vi "MoveAwayFromBallSkill.vi"(8 "error in (no error)":errorcluster, 9 "Game in":refnum<class "Game.lvclass">, 10 "Robot":refnum<class "Robot.lvclass">, 11 "MoveAwayFromBallSkill in":refnum<class "MoveAwayFromBallSkill.lvclass">) -> (0 "error out":errorcluster, 2 "Robot out":refnum<class "Robot.lvclass">, 3 "MoveAwayFromBallSkill out":refnum<class "MoveAwayFromBallSkill.lvclass">)   [LabVIEW 2023, in "MoveAwayFromBallSkill.lvclass"]
uses:
  MoveAwayFromBallSkill.lvclass
  Robot_class/Robot.lvclass
  C:/Users/lucio/Desktop/roboime/SSL_AI/Object_class/Object.lvclass
  Game_class/Game.lvclass
  Game_class/Game.lvclass/Game.ctl
  Parameters_class/Parameters.lvclass/Parameters.ctl
  Object_class/Object.lvclass/Object.ctl
  Robot_class/Robot.lvclass/Robot.ctl
  <vilib>/Analysis/baseanly.llb/Unit Vector (DBL).vi
  Object_class/Read position(x,y).vi
  Game_class/Read Parameters.lvclass.vi
  Game_class/Read BallRef.vi
  Parameters_class/Read DistanceStop.vi
  Robot_class/Write dest_x.vi
  Robot_class/Write dest_y.vi
  Robot_class/Write dest_orientation.vi
  Ball_class/Ball.lvclass
  Parameters_class/Parameters.lvclass
  <vilib>/Analysis/NI_AALBase.lvlib
  Utilities_class/Utilities.lvclass
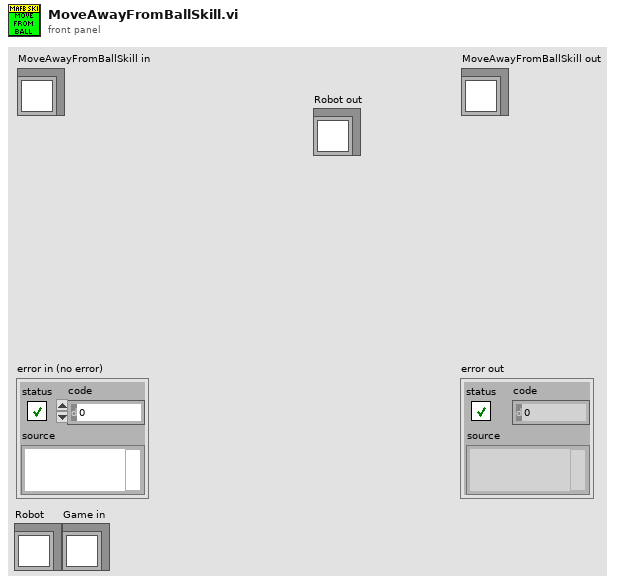
[diagram p1: front panel]
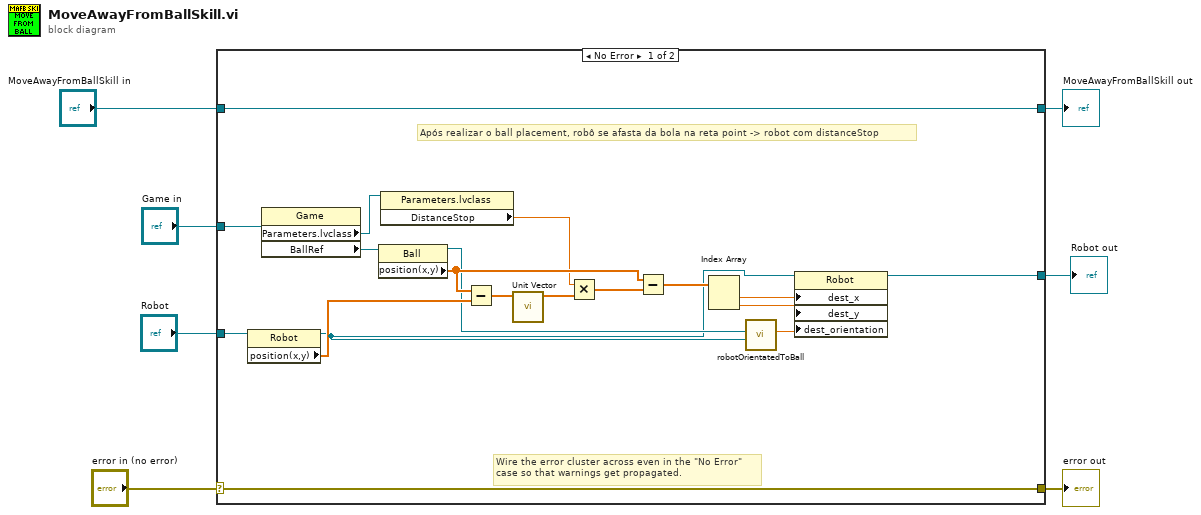
[diagram p0: block diagram]
diagram:
  n1 = case shown="No Error" "error in (no error)" {
    selector: "error in (no error)" -> [w25 w28]
    tunnel: [w25 w28] -> w6
    tunnel: [w26 w27] -> w4
    tunnel: "MoveAwayFromBallSkill in" -> [w26 w27]
    tunnel: "Game in" -> [w24 _]
    tunnel: "Robot" -> [w15 _]
    tunnel: [w11 _] -> w1
    frame No Error {
      # "Após realizar o ball placement, robô se afasta da bola na reta point -> robot com distanceStop"
      # "Wire the error cluster across even in the \"No Error\"\ncase so that warnings get propagated."
      n2 = property class="Robot"(reference=w15) -> (reference out=w8:refnum<class "Robot.lvclass">, "position(x,y)"=w22:dbl[])  [unwired: 1 in, 1 out]
      n3 = property class="Game"(reference=w24) -> ("Parameters.lvclass"=w18:refnum<class "Parameters.lvclass">, "BallRef"=w23:refnum<class "Ball.lvclass">)  [unwired: 1 in, 2 out]
      n4 = property class="Ball"(reference=w23) -> (reference out=w9:refnum<class "Ball.lvclass">, "position(x,y)"=w21:dbl[])  [unwired: 1 in, 1 out]
      n5 = property class="Parameters.lvclass"(reference=w18) -> ("DistanceStop"=w17:dbl)  [unwired: 1 in, 2 out]
      n6 = Subtract(x=w21, y=w22) -> (x-y=w20:dbl[])
      n7 = call-poly <vilib>:"Unit Vector.vi"("Input Vector"=w20) -> ("Unit Vector"=w19:dbl[])  [unwired: 8 in, 2 out]
      n8 = Multiply(x=w17, y=w19) -> (x*y=w16:dbl[])
      n9 = Subtract(x=w21, y=w16) -> (x-y=w14:dbl[])
      n10 = Index Array(array=w14) -> (element #1=w13:dbl, element #2=w12:dbl)  [unwired: 2 in]
      n11 = call "robotOrientatedToBall.vi"("Robot"=w8, "BallRef"=w9) -> ("Orientation"=w10:dbl)  [unwired: 7 in, 2 out]
      n12 = property class="Robot"(reference=w8, "dest_x"=w13, "dest_y"=w12, "dest_orientation"=w10) -> (reference out=w11:refnum<class "Robot.lvclass">)  [unwired: 1 in, 1 out]
    }
    frame Error {
    }
  }
  "error out" <- w6
  "MoveAwayFromBallSkill out" <- w4
  "Robot out" <- w1
